vi "LightControl.vi"(8 "error in (no error)":errorcluster, 10 "X":dbl, 11 "Boolean":bool) -> (0 "error out":errorcluster)   [LabVIEW 2015]
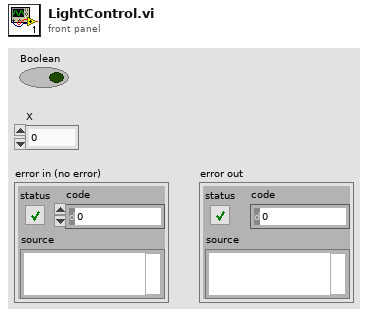
[diagram p1: front panel]
types:
  T1 = cluster{"Boolean":bool, "intensity":u8, "flashspeed":u8, "intensity":u8, "flashspeed":u8}
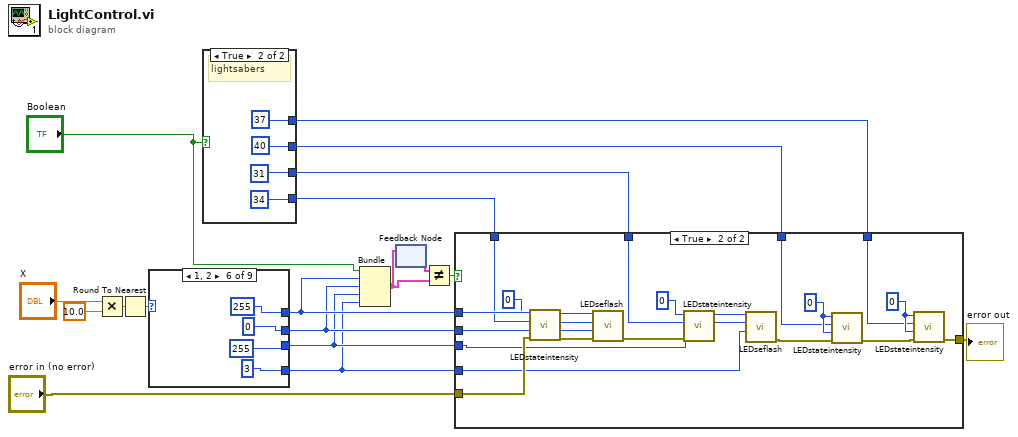
[diagram p0: block diagram]
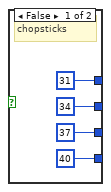
[diagram p3: hidden frame]
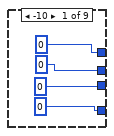
[diagram p4: hidden frame]
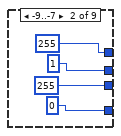
[diagram p5: hidden frame]
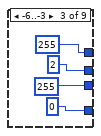
[diagram p6: hidden frame]
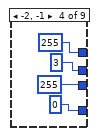
[diagram p7: hidden frame]
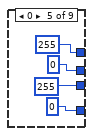
[diagram p8: hidden frame]
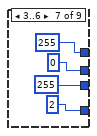
[diagram p9: hidden frame]
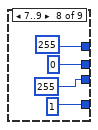
[diagram p10: hidden frame]
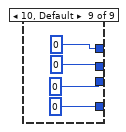
[diagram p11: hidden frame]
diagram:
  n1 = Multiply(x="X", y=10.0) -> (x*y=w4:dbl)
  n2 = Round To Nearest(number=w4) -> (nearest integer value=w10:dbl)
  n3 = case shown="1, 2" w10 {
    tunnel: [u8 0 ("flashspeed") u8 1 ("flashspeed") u8 2 ("flashspeed") u8 3 ("flashspeed") u8 0 ("flashspeed") u8 0 ("flashspeed") u8 0 ("flashspeed") u8 0 ("flashspeed") u8 0 ("flashspeed")] -> w13
    tunnel: [u8 0 ("intensity") u8 255 ("intensity") u8 255 ("intensity") u8 255 ("intensity") u8 255 ("intensity") u8 255 ("intensity") u8 255 ("intensity") u8 255 ("intensity") u8 0 ("intensity")] -> w14
    tunnel: [u8 0 ("flashspeed") u8 0 ("flashspeed") u8 0 ("flashspeed") u8 0 ("flashspeed") u8 0 ("flashspeed") u8 3 ("flashspeed") u8 2 ("flashspeed") u8 1 ("flashspeed") u8 0 ("flashspeed")] -> w11
    tunnel: [u8 0 ("intensity") u8 255 ("intensity") u8 255 ("intensity") u8 255 ("intensity") u8 255 ("intensity") u8 255 ("intensity") u8 255 ("intensity") u8 255 ("intensity") u8 0 ("intensity")] -> w12
    frame -10 {
    }
    frame -9..-7 {
    }
    frame -6..-3 {
    }
    frame -2, -1 {
    }
    frame 0 {
    }
    frame 1, 2 {
    }
    frame 3..6 {
    }
    frame 7..9 {
    }
    frame 10, Default {
    }
  }
  n4 = case shown="True" "Boolean" {
    tunnel: [i16 31 ("port") i16 37 ("port")] -> w6
    tunnel: [i16 34 ("port") i16 40 ("port")] -> w7
    tunnel: [i16 37 ("port") i16 31 ("port")] -> w8
    tunnel: [i16 40 ("port") i16 34 ("port")] -> w9
    frame False {
      # "chopsticks"
    }
    frame True {
      # "lightsabers"
    }
  }
  n5 = Bundle("Boolean"="Boolean", "intensity"=w14, "flashspeed"=w13, "intensity"=w12, "flashspeed"=w11) -> (w17:T1)  [unwired: 1 in]
  n6 = feedback #1() -> (w18:T1)  [unwired: 1 in]
  n7 = feedback-in #1(w17) -> ()
  n8 = Not Equal?(x=w18, y=w17) -> (x != y?=w16:bool)
  n9 = case shown="True" w16 {
    tunnel: w13 -> [_ w83]
    tunnel: w14 -> [_ w81]
    tunnel: "error in (no error)" -> [w63 w80]
    tunnel: w11 -> [_ w75]
    tunnel: [w63 w71] -> w5
    tunnel: w6 -> [_ w68]
    tunnel: w7 -> [_ w67]
    tunnel: w8 -> [_ w66]
    tunnel: w9 -> [_ w65]
    tunnel: w12 -> [_ w64]
    frame False {
    }
    frame True {
      w70 = i16 0 ("Id")
      w69 = i16 0 ("Id")
      n10 = call "LEDstateintensity.vi"("error in (no error)"=w80, "intensity"=w81, "port"=w65, "Id"=i16 0) -> ("error out"=w82:errorcluster, "port out"=w85:i16, "Id out"=w84:i16)  [unwired: 5 in]
      n11 = call "LEDseflash.vi"("error in (no error)"=w82, "flashspeed"=w83, "port"=w85, "Id"=w84) -> ("error out"=w74:errorcluster)  [unwired: 7 in]
      n12 = call "LEDstateintensity.vi"("error in (no error)"=w74, "intensity"=w64, "port"=w66, "Id"=i16 0) -> ("port out"=w76:i16, "Id out"=w77:i16)  [unwired: 5 in, 1 out]
      n13 = call "LEDseflash.vi"("flashspeed"=w75, "port"=w76, "Id"=w77) -> ("error out"=w73:errorcluster)  [unwired: 8 in]
      n14 = call "LEDstateintensity.vi"("error in (no error)"=w73, "intensity"=w69, "port"=w67, "Id"=w69) -> ("error out"=w72:errorcluster)  [unwired: 5 in, 2 out]
      n15 = call "LEDstateintensity.vi"("error in (no error)"=w72, "intensity"=w70, "port"=w68, "Id"=w70) -> ("error out"=w71:errorcluster)  [unwired: 5 in, 2 out]
    }
  }
  "error out" <- w5
